vi "rename channel in mapping.vi"(7 "owner ID":string, 8 "error in":errorcluster, 9 "new channel":refnum<class "TBM channel.lvclass">, 10 "old channel":refnum<class "TBM channel.lvclass">, 11 "engine configuration in":refnum<class "engine configuration.lvclass">) -> (0 "error out":errorcluster, 3 "engine configuration out":refnum<class "engine configuration.lvclass">)   [LabVIEW 2013, in "engine configuration.lvclass"]
doc: "This function renames a mapped channel specified by 'old channel' with the new name specified in 'new channel'."
uses:
  engine configuration.lvclass
  <vilib>/NI/Tag Bus Module Framework/channel/TBM channel.lvclass
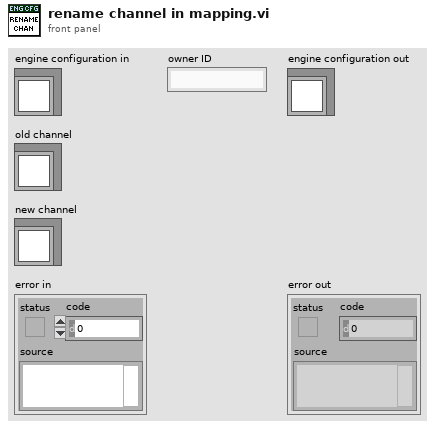
[diagram p1: front panel]
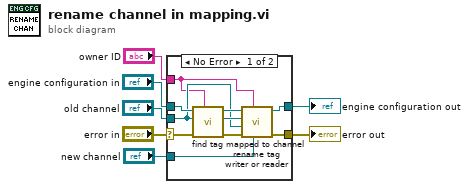
[diagram p0: block diagram]
diagram:
  n1 = case shown="No Error" "error in" {
    selector: "error in" -> [w12 w19]
    tunnel: [w16 w19] -> w6
    tunnel: [w15 w18] -> w4
    tunnel: "engine configuration in" -> [w14 w18]
    tunnel: "owner ID" -> [w8 _]
    tunnel: "old channel" -> [w9 _]
    tunnel: "new channel" -> [w17 _]
    frame No Error {
      n2 = call "find tag mapped to channel.vi"("owner"=w8, "error in"=w12, "channel"=w9, "engine configuration in"=w14) -> ("error out"=w11:errorcluster, "tag"=w10:refnum<class "tag descriptor.lvclass">, "engine configuration out"=w13:refnum<class "engine configuration.lvclass">)  [unwired: 5 in]
      n3 = call "rename tag writer or reader.vi"("new channel"=w17, "owner ID"=w8, "error in"=w11, "old channel"=w9, "tag descriptor"=w10, "engine configuration in"=w13) -> ("error out"=w16:errorcluster, "engine configuration out"=w15:refnum<class "engine configuration.lvclass">)  [unwired: 4 in]
    }
    frame Error {
    }
  }
  "error out" <- w6
  "engine configuration out" <- w4
